vi "Read MVA Object In Terminal.vi"(8 "error in (no error)":errorcluster, 11 "MVA Comms VI Instance in":refnum<class "MVA Comms VI Instance.lvclass">) -> (0 "error out":errorcluster, 2 "MVA Object In Terminal":i32=10, 3 "MVA Comms VI Instance out":refnum<class "MVA Comms VI Instance.lvclass">)   [LabVIEW 2020, in "MVA Message Mapper.lvlib" / "MVA Comms VI Instance.lvclass"]
uses:
  <vilib>/gpm_packages/@cs/Bus-message-mapper/Source/support/MVA Comms/MVA Comms VI Instance.lvclass
  <vilib>/gpm_packages/@cs/Bus-message-mapper/Source/support/MVA Comms/MVA Comms VI Instance.lvclass/MVA Comms VI Instance.ctl
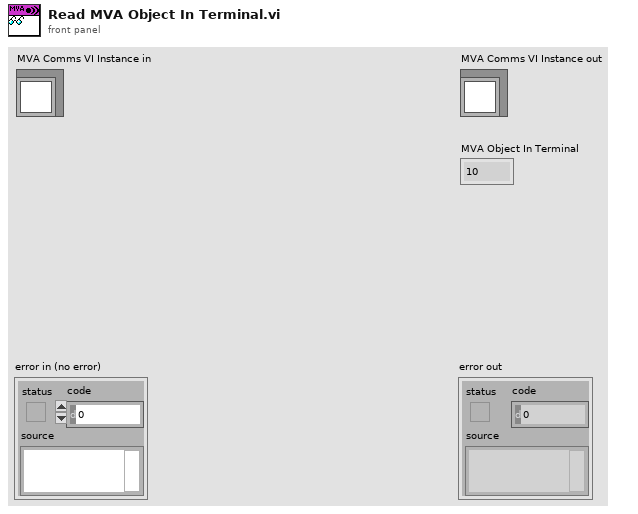
[diagram p1: front panel]
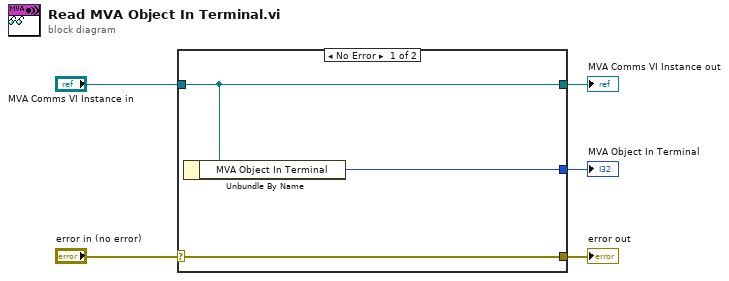
[diagram p0: block diagram]
diagram:
  n1 = case shown="No Error" "error in (no error)" {
    selector: "error in (no error)" -> [w8 w9]
    tunnel: [w8 w9] -> w4
    tunnel: [w7 w10] -> w2
    tunnel: "MVA Comms VI Instance in" -> [w7 w10]
    tunnel: [w6 _] -> w1
    frame No Error {
      n2 = Unbundle By Name(w7) -> ("MVA Object In Terminal"=w6:i32)
    }
    frame Error {
    }
  }
  "error out" <- w4
  "MVA Comms VI Instance out" <- w2
  "MVA Object In Terminal" <- w1
